vi "Align.vi"(8 "Command Info In":T1, 11 "Auto Align":bool) -> (0 "Command Info Out":T1)   [LabVIEW 2020]
uses:
  <vilib>/Rock Robotics/WPI/Framework/Command Status Info.ctl
  <vilib>/Rock Robotics/WPI/Framework/Completion Status.ctl
  <vilib>/Rock Robotics/WPI/Framework/Completion Notifier.ctl
  Framework/Robot Global Data.vi
  <vilib>/Rock Robotics/Network Tables/NT Write Number.vi
  <vilib>/Rock Robotics/Network Tables/NT Write Boolean.vi
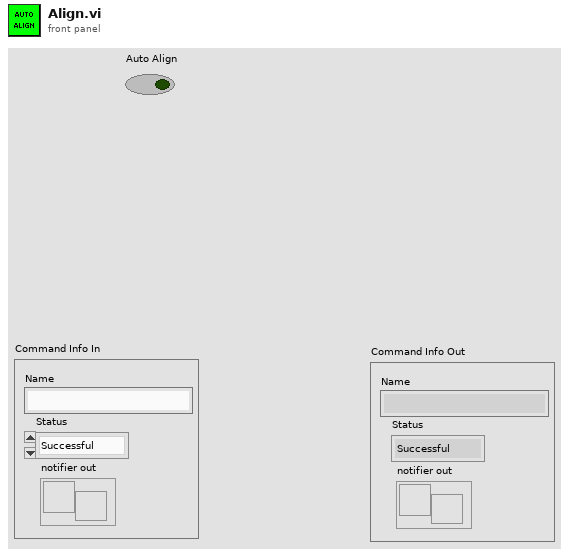
[diagram p1: front panel]
types:
  T1 = typedef "Command Status Info.ctl" = cluster{"Name":string, "Status":T2, "notifier out":T3}
  T2 = typedef "Completion Status.ctl" = enum16{"Successful", "Aborted", "Incomplete"}
  T3 = typedef "Completion Notifier.ctl" = refnum<notifier>
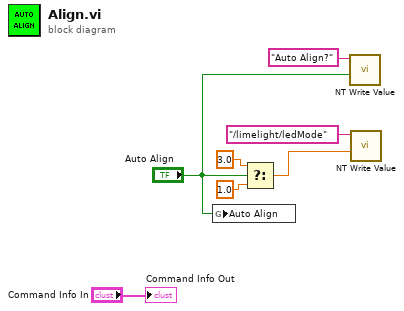
[diagram p0: block diagram]
diagram:
  n1 = global write "Robot Global Data.vi" "Auto Align"("Auto Align") -> ()
  n2 = Select(t=3.0 ("Numeric"), s="Auto Align", f=1.0) -> (s? t:f=w4:dbl)
  n3 = call-poly <vilib>:"NT Write Value.vi"("Boolean"="Auto Align", "Name"="Auto Align?") -> ()  [unwired: 9 in, 1 out]
  n4 = call-poly <vilib>:"NT Write Value.vi"("Numeric"=w4, "Name"="/limelight/ledMode") -> ()  [unwired: 9 in, 1 out]
  "Command Info Out" <- "Command Info In"
